vi "2ndOrderDiffEqnPolarCoeffs.vi"(6 "Enable?":bool, 9 "Theta":fxp<+/-,24,1>, 10 "r":fxp<+/-,24,1>, 11 "Input":fxp<+/-,18,5>) -> (3 "Output":fxp<+/-,18,5>)   [LabVIEW 2019]
doc: "Implement a first order difference equation of the form:\ny(k) = 2*r*cos(Theta)*y(k-1) + (r^2)*y(k-2) + (1- 2*r*cos(Theta)-(r^2))*u(k)\n\nSet values of r such that (0<=r<=1) and Theta such that (-180<=Theta<=180) degrees.\n\nDropped the idea to make these calculations in the RT target and then Send to FPGA with the regular 2nd Order Diff. Eqn. VI."
uses:
  <vilib>/Platform/TimedLoop/XDataNode/XDataNode.xnode
  <vilib>/Platform/TimedLoop/XDataNode/nitl_modes.ctl
  <vilib>/Platform/TimedLoop/XDataNode/XDNodeRunTimeDep.lvlib
  <vilib>/Platform/TimedLoop/XDataNode/wakeup.ctl
  <vilib>/Platform/TimedLoop/XDataNode/timing_clust.ctl
  <vilib>/rvi/FXPMathLib/FxpMul/XNode/nifxpmath_Multiplier.xnode
  <vilib>/rvi/FXPMathLib/sim/FxpSim.dll
  <vilib>/rvi/FXPMathLib/FxpSub/XNode/nifxpmath_Sub.xnode
  <vilib>/rvi/FXPMathLib/FxpAdd/XNode/nifxpmath_Add.xnode
  <vilib>/rvi/FXPMathLib/FxpSinAndCos/XNode/nifxpmath_SinAndCos.xnode
  <vilib>/rvi/FXPMathLib/FxpSinAndCos/simVIs/DllFxpSinAndCosTemp_sub.vi
  <vilib>/rvi/FXPMathLib/FxpSinAndCos/subVIs/nifxpmath_SinAndCos_SimConfig.ctl
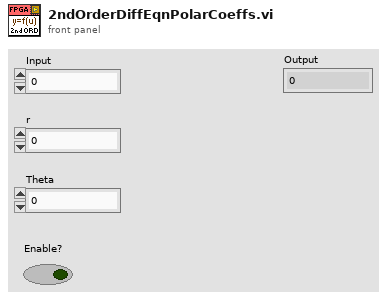
[diagram p1: front panel]
types:
  T1 = typedef "XDNodeRunTimeDep.lvlib/timing_clust.ctl" = cluster{"Expected End [f-1]":u64, "Actual End [f-1]":u64, "Finished Late? [f-1]":bool, "Expected End [i-1]":u64, "Actual End [i-1]":u64, "Finished Late? [i-1]":bool, "Expected Start [i]":u64, "Actual Start [i]":u64, "Expected Start [f]":u64, "Actual Start [f]":u64, "Source Name":string, "Structure Name":string, "Period":i64, "Deadline":i64, "Offset":i64, "Start":i64, "Priority":i32, "Timeout":i32, "Mode":T2, "Wakeup Reason":T3, "Error":errorcluster, "Source Type":string, "Secondary Source Type":string, "Global End Time":u64, "Global Start Time":u64, "Frame Duration":u64, "Iteration Duration":u64, "Assigned CPU":i32, "I/O Scan Engine Mode":u32}
  T2 = typedef "XDNodeRunTimeDep.lvlib/nitl_modes.ctl" = enum32{"No Change", "Process missed periods, maintain original phase", "Discard missed periods, maintain original phase", "Process missed periods, ignore original phase", "Discard missed periods, ignore original phase"}
  T3 = typedef "XDNodeRunTimeDep.lvlib/wakeup.ctl" = enum32{"Normal", "Aborted", "Asynchronous wakeup", "Timing source error", "Timed loop error", "Timeout"}
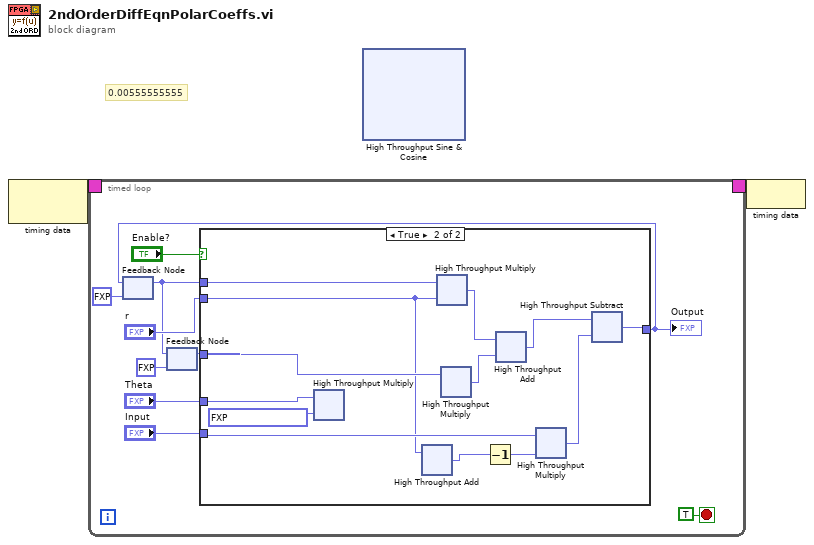
[diagram p0: block diagram]
diagram:
  # "0.00555555555"
  n1 = node-c288() -> (w2:T1)  [unwired: 1 in]
  n2 = timed-loop {
    timing: w2 -> [_]
    timing-out: [_] -> w1
    stop <- TRUE stop-if-true
    n3 = feedback #1(fxp<+/-,18,5> 0.0 ("x+y")) -> (w5:fxp<+/-,18,5>)
    n4 = feedback #2(fxp<+/-,18,5> 0.0 ("x+y")) -> (w4:fxp<+/-,18,5>)
    n5 = feedback-in #2(w5) -> ()
    n6 = case shown="True" "Enable?" {
      tunnel: "Input" -> [w13 w25]
      tunnel: "r" -> [_ w19]
      tunnel: [w13 w24] -> w8
      tunnel: w5 -> [_ w23]
      tunnel: w4 -> [_ w21]
      tunnel: "Theta" -> [_ w15]
      frame False {
      }
      frame True {
        n7 = xnode "High Throughput Multiply"("x"=w15, "y"=fxp<+/-,16,1> 0.00555419921875) -> ()  [unwired: 1 out]
        n8 = xnode "High Throughput Add"("x"=w19) -> ("x+y"=w20:fxp<+/-,25,2>)  [unwired: 1 in]
        n9 = xnode "High Throughput Multiply"("x"=w23, "y"=w19) -> ("x*y"=w17:fxp<+/-,18,5>)
        n10 = xnode "High Throughput Multiply"("x"=w21) -> ("x*y"=w18:fxp<+/-,18,5>)  [unwired: 1 in]
        n11 = Decrement(x=w20) -> (x-1=w22:fxp<+/-,26,3>)
        n12 = xnode "High Throughput Add"("x"=w17, "y"=w18) -> ("x+y"=w16:fxp<+/-,19,6>)
        n13 = xnode "High Throughput Multiply"("x"=w25, "y"=w22) -> ("x*y"=w26:fxp<+/-,18,5>)
        n14 = xnode "High Throughput Subtract"("x"=w16, "y"=w26) -> ("x-y"=w24:fxp<+/-,18,5>)
      }
    }
    "Output" <- w8
    n15 = feedback-in #1(w8) -> ()
  }
  n16 = xnode "High Throughput Sine & Cosine"() -> ()  [unwired: 1 in, 2 out]
  n17 = node-c288(w1) -> ()
